vi "arrays_clusters_bundles.vi"() -> ()   [LabVIEW 2014]
panel:
  in  "Cluster Control 2":T1
  out "cluster2 num":dbl
  out "cluster2 bool":bool
  out "cluster2 string":string
  out "cluster1 string":string
  out "cluster1 bool":bool
  out "cluster1 num":dbl
  in  "length2":i32
  in  "index2":i32
  in  "length1":i32
  in  "index1":i32
  out "subarray":dbl[][](array[numeric])
  in  "Predefined Array":dbl[][](array[numeric])=[[1.0, 2.0, 3.0], [4.0, 5.0, 6.0]]
  out "Cluster Indicator":T2
  in  "Cluster Control":T2
  in  "dimension size (Column)":i32=3
  in  "dimension size (Row)":i32=2
  in  "Initial Value":dbl
  out "Array Indicator 2":dbl[][](array[numeric])
  out "Array Indicator":dbl[](array[numeric])
  in  "Array Control":dbl[](array[numeric])
  # "1-D Array"
  # "2-D Array"
  # "Row"
  # "Col"
  # "Clusters"
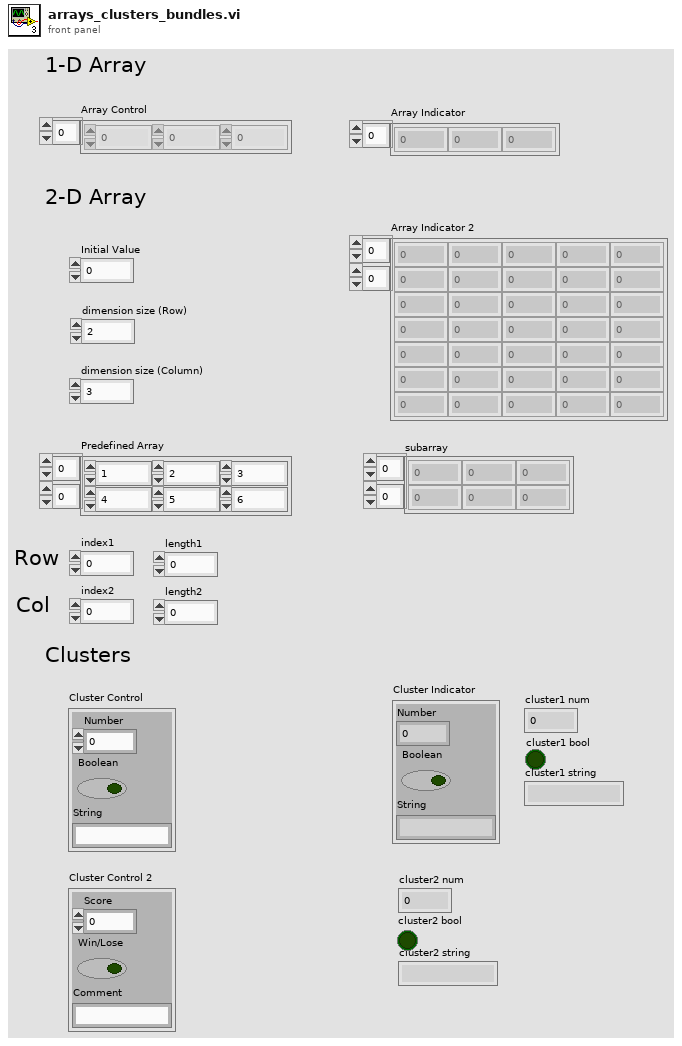
[diagram p1: front panel]
types:
  T1 = cluster{"Score":dbl, "Win/Lose":bool, "Comment":string}
  T2 = cluster{"Number":dbl, "Boolean":bool, "String":string}
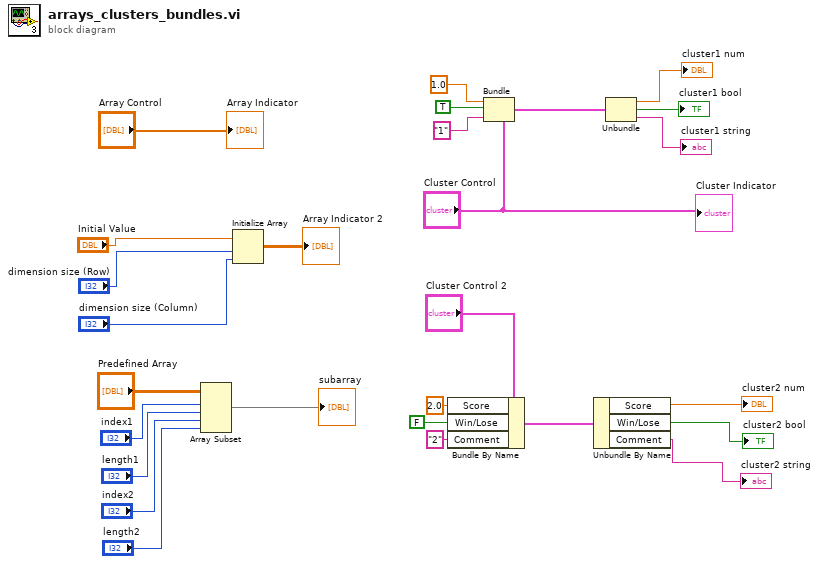
[diagram p0: block diagram]
diagram:
  n1 = Array Subset(array="Predefined Array", index (row)="index1", length (row)="length1", index (col)="index2", length (col)="length2") -> (→"subarray":dbl[][])
  n2 = Initialize Array("Initial Value", "dimension size (Row)", "dimension size (Column)") -> (→"Array Indicator 2":dbl[][])
  n3 = Bundle By Name(cluster="Cluster Control 2", "Score"=2.0 ("Number"), "Win/Lose"=FALSE ("Boolean"), "Comment"="2" ("String")) -> (w15:T1)
  n4 = Bundle(cluster="Cluster Control", "Number"=1.0, "Boolean"=TRUE, "String"="1") -> (w14:T2)
  n5 = Unbundle By Name(w15) -> ("Score"=→"cluster2 num":dbl, "Win/Lose"=→"cluster2 bool":bool, "Comment"=→"cluster2 string":string)
  n6 = Unbundle(w14) -> ("Number"=→"cluster1 num":dbl, "Boolean"=→"cluster1 bool":bool, "String"=→"cluster1 string":string)
  "Array Indicator" <- "Array Control"
  "Cluster Indicator" <- "Cluster Control"
